vi "Logger.vi"(6 "Verbose (T)":bool=TRUE, 7 "Log Type (System)":T1, 9 "CR/LF? (T)":bool=TRUE, 10 "Information":string, 11 "Action (Append)":enum16{"Init", "Read", "Append", "Save to File"}(ring)=enum."Append") -> (0 "error out":errorcluster, 1 "Data Log":string, 2 "System Log":string, 3 "Error Log":string)   [LabVIEW 2011]
doc: "Maintains logging information in a simple functional global.\n\nThree logs are maintained for flexibility with System Log being the default.\n\n<b>Log</b> - Specifies to use System, Error or Data Log for current operation.\n\n<b>Action</b>:\n - Init - Initialize the Log with Information string passed in.\n - <b>Append</b>\n - Read - Return current Log.\n - Save to File - save the current Log to the file specified by the Information input.\n\n<b>EOL?</b> - Appends an EOL character when adding to the Log.\n\n<b>Information</b> - Information to add to the Log (Init, Append) or path to log file (Save to File).\n\n<b>Log</b> - Current value of the Log.\n\n\nVersion 1.2 - 6/1/2010\n\nPhaeron, Inc.\nwww.phaeron.com\ninfo@phaeron.com"
uses:
  Log Type.ctl
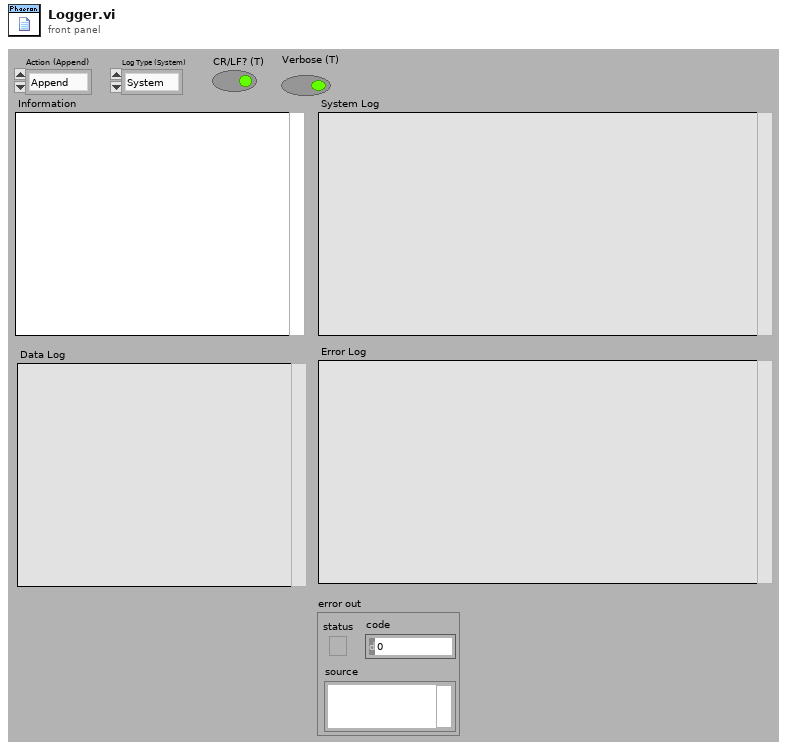
[diagram p1: front panel]
types:
  T1 = typedef "Log Type.ctl" = enum16{"System", "Data", "Error"}
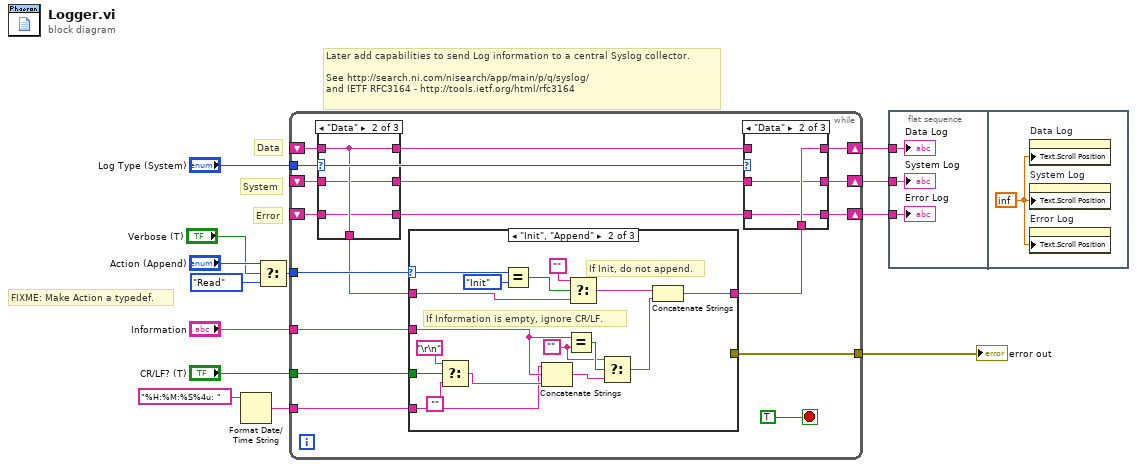
[diagram p0: block diagram]
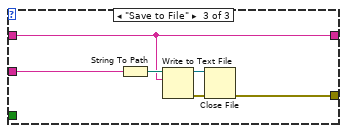
[diagram p7: hidden frame]
diagram:
  # "FIXME: Make Action a typedef."
  # "Error"
  # "Later add capabilities to send Log information to a central Syslog collector.\n\nSee http://search.ni.com/nisearch/app/main/p/q/syslog/\nand IETF RFC3164 - http://tools.ietf.org/html/rfc3164"
  # "System"
  # "Data"
  n1 = Format Date/Time String(time format string (%c)="%H:%M:%S%4u: ") -> (date/time string=w5:string)  [unwired: 2 in]
  n2 = Select(t="Action (Append)", s="Verbose (T)", f=enum16{"Init", "Read", "Append", "Save to File"}."Read") -> (s? t:f=w4:enum16{"Init", "Read", "Append", "Save to File"})
  n3 = while {
    tunnel: w4 -> [w30]
    shift-right: [w19] -> w10
    shift-left: _ -> [w25]
    tunnel: [w29] -> w13
    tunnel: "Information" -> [w28]
    tunnel: "CR/LF? (T)" -> [w27]
    shift-right: [w18] -> w9
    shift-left: _ -> [w26]
    tunnel: "Log Type (System)" -> [w23]
    shift-right: [w17] -> w7
    shift-left: _ -> [w15]
    tunnel: w5 -> [w14]
    stop <- TRUE stop-if-true
    n4 = case shown="\"Data\"" w23 {
      tunnel: w26 -> [w42 w46 w48]
      tunnel: w25 -> [w43 w45 w49]
      tunnel: [w43 w46 w47] -> w24
      tunnel: [w43 w45 w49] -> w22
      tunnel: [w42 w46 w48] -> w21
      tunnel: [w41 w44 w47] -> w16
      tunnel: w15 -> [w41 w44 w47]
      frame "System", Default {
      }
      frame "Data" {
      }
      frame "Error" {
      }
    }
    n5 = case shown="\"Init\", \"Append\"" w30 {
      selector: w30 -> [_ w63 _]
      tunnel: [w50 w53 w71] -> w20
      tunnel: w24 -> [w50 w52 w71]
      tunnel: w28 -> [_ w56 w72]
      tunnel: [_ _ w68] -> w29
      tunnel: w27 -> [_ w66 _]
      tunnel: w14 -> [_ w51 _]
      frame "Read", Default {
      }
      frame "Init", "Append" {
        w58 = ""
        # "If Information is empty, ignore CR/LF."
        # "If Init, do not append."
        n6 = Select(t="\r\n", s=w66, f="") -> (s? t:f=w55:string)
        n7 = Equal?(x=w63, y=enum16{"Init", "Read", "Append", "Save to File"}."Init") -> (x = y?=w64:bool)
        n8 = Concatenate Strings(w51, w56, w55) -> (w54:string)
        n9 = Equal?(x=w56, y=w58) -> (x = y?=w59:bool)
        n10 = Select(t="", s=w64, f=w52) -> (s? t:f=w61:string)
        n11 = Select(t=w58, s=w59, f=w54) -> (s? t:f=w57:string)
        n12 = Concatenate Strings(w61, w57) -> (w53:string)
      }
      frame "Save to File" {
        n13 = String To Path(string=w72) -> (path=w73:path)
        n14 = Write to Text File(file (use dialog)=w73, text=w71) -> (refnum out=w69:refnum<file>, error out=w70:errorcluster)  [unwired: 2 in, 1 out]
        n15 = Close File(refnum=w69, error in=w70) -> (error out=w68:errorcluster)  [unwired: 1 out]
      }
    }
    n16 = case shown="\"Data\"" w23 {
      tunnel: w21 -> [w33 _ w38]
      tunnel: w22 -> [_ w36 w39]
      tunnel: w20 -> [w34 w37 w40]
      tunnel: [w34 w36 w39] -> w19
      tunnel: [w33 w37 w38] -> w18
      tunnel: [w32 w35 w40] -> w17
      tunnel: w16 -> [w32 w35 _]
      frame "System", Default {
      }
      frame "Data" {
      }
      frame "Error" {
      }
    }
  }
  "error out" <- w13
  n17 = flat-sequence {
    tunnel: w10 -> [w76]
    tunnel: w9 -> [w75]
    tunnel: w7 -> [w74]
    frame #0 {
      "System Log" <- w76
      "Data Log" <- w75
      "Error Log" <- w74
    }
    frame #1 {
      w77 = inf
      n18 = property on="Data Log" class="Str"("Text.Scroll Position"=w77) -> ()  [unwired: 2 in, 2 out]
      n19 = property on="System Log" class="Str"("Text.Scroll Position"=w77) -> ()  [unwired: 2 in, 2 out]
      n20 = property on="Error Log" class="Str"("Text.Scroll Position"=w77) -> ()  [unwired: 2 in, 2 out]
    }
  }
